vi "Read Config.vi"(8 "error in (no error)":errorcluster, 10 "Path to Config Folder":path, 11 "Fixture Config in":refnum<class "Fixture Config.lvclass">) -> (0 "error out":errorcluster, 3 "Fixture Config out":refnum<class "Fixture Config.lvclass">)   [LabVIEW 2017, in "Station Config.lvlib" / "Fixture Config.lvclass"]
doc: "Reads a recipe for a specified Material Type and stores it into memory."
uses:
  Fixture Config.lvclass
  Class/Station Config.lvclass
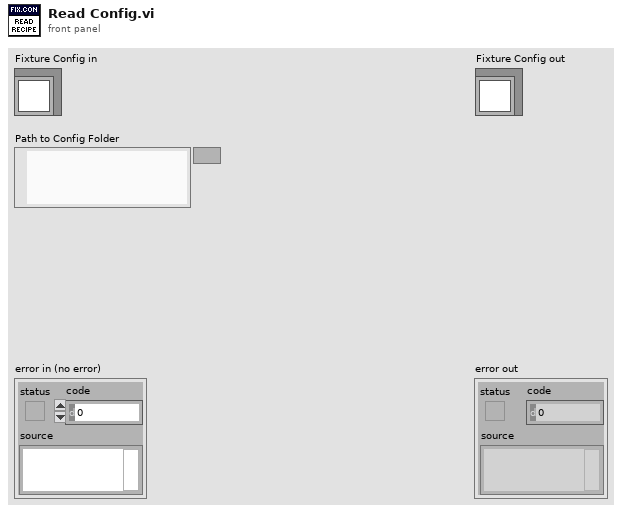
[diagram p1: front panel]
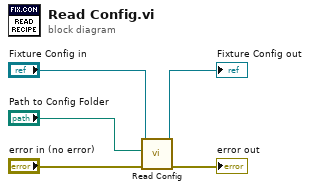
[diagram p0: block diagram]
diagram:
  n1 = call-parent "Read Config.vi"("error in (no error)"="error in (no error)", "Path to Config Folder"="Path to Config Folder", "Station Config in"="Fixture Config in") -> ("error out"=→"error out":errorcluster, "Station Config out"=→"Fixture Config out":refnum<class "Fixture Config.lvclass">)  [unwired: 7 in]
